vi "CalcRearLeft.vi"(9 "Rotate Clockwise\n(Input)":dbl, 10 "Strafe Left\n(Input)":dbl, 11 "Forward\n(Input)":dbl format="%#_13g") -> (2 "Motor Speed\n(Output)":dbl)   [LabVIEW 2014]
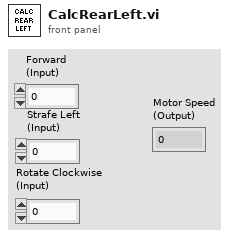
[diagram p1: front panel]
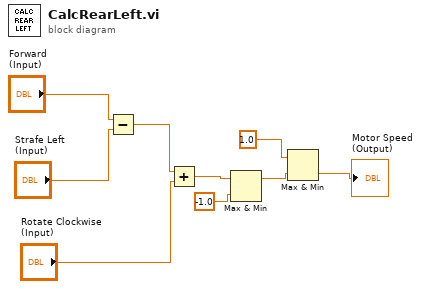
[diagram p0: block diagram]
diagram:
  n1 = Subtract(x="Forward\n(Input)", y="Strafe Left\n(Input)") -> (x-y=w6:dbl)
  n2 = Add(x=w6, y="Rotate Clockwise\n(Input)") -> (x+y=w5:dbl)
  n3 = Max & Min(x=w5, y=-1.0) -> (max(x,y)=w3:dbl)  [unwired: 1 out]
  n4 = Max & Min(x=1.0, y=w3) -> (min(x,y)=→"Motor Speed\n(Output)":dbl)  [unwired: 1 out]
